vi "LCA Get Actual Postition XY.vi"(8 "error in (no error)":errorcluster caption="Fehler (Eingang, kein Fehler)", 11 "Axis System Handle":i64) -> (0 "error out":errorcluster caption="Fehler (Ausgang)", 2 "Position Y":dbl, 3 "Position X":dbl)   [LabVIEW 2021, in "labbCAN_MotionControl_API.lvlib"]
doc: "LCA_Func long __stdcall LCA_GetActualPostitionXY(dev_hdl hAxisSystem,\n double* pfPosIsX,\n double* pfPosIsY);"
uses:
  labbCAN_MotionControl_API.lvlib
  labbCAN_MotionControl_API.dll
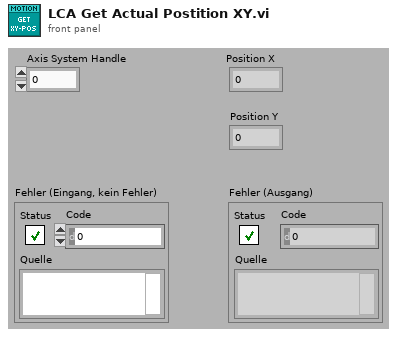
[diagram p1: front panel]
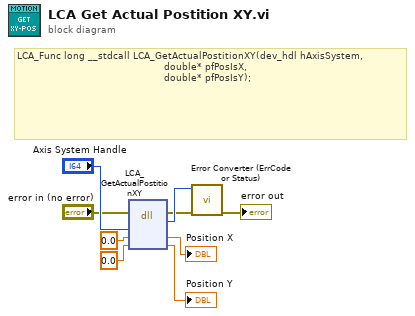
[diagram p0: block diagram]
diagram:
  # "LCA_Func long __stdcall LCA_GetActualPostitionXY(dev_hdl hAxisSystem,\n                                                 double* pfPosIsX,\n                                                 double* pfPosIsY);"
  n1 = dll-call lib="C:/Users/olaja/AppData/Local/CETONI_SDK/labbCAN_MotionControl_API.*" fn="LCA_GetActualPostitionXY"(error in="error in (no error)", "hAxisSystem"="Axis System Handle", "pfPosIsX"=0.0, "pfPosIsY"=0.0) -> (error out=w2:errorcluster, "Rückgabetyp"=w3:i32, "pfPosIsX"=→"Position X":dbl, "pfPosIsY"=→"Position Y":dbl)  [unwired: 3 in, 1 out]
  n2 = call "Error Converter (ErrCode or Status).vi"("error in (no error)"=w2, "error code"=w3) -> ("error out"=→"error out":errorcluster)  [unwired: 9 in]
